vi "prepAI_tt.vi"   [LabVIEW 2013]
uses:
  <vilib>/DAQmx/create/channels.llb/DAQmx Create Channel (AI-Voltage-Basic).vi
  <vilib>/DAQmx/configure/timing.llb/DAQmx Timing (Sample Clock).vi
types:
  T1 = cluster{"StageS":i32, "StageL":i32, "data dir":path, "image OD":u16, "contour OD":u16, "point OD":u16, "AOlines":tag[], "AIlines":tag[], "CI lines":tag[], "DO lines":tag[], "AO names":string[], "CI names":string[], "AI names":string[], "DO names":string[], "CIextensions":string[], "AIextensions":string[], "Voltage to Ygalvo":i32, "Voltage to Xgalvo":i32, "Voltage to patch":i32, "640 shutter":i32, "2P shutter":i32, "LT timestamp":i32}
  T2 = typedef "LVRectTypeDef.ctl" = cluster{"Left":i16, "Top":i16, "Right":i16, "Bottom":i16}
  T3 = cluster{"Xpixels":i32, "Vxminref":dbl, "Vxmaxref":dbl, "P":dbl, "Ypixels":i32, "Vyminref":dbl, "Vymaxref":dbl, "srate":sgl, "sAOxy":i32, "timeout":dbl, "type":string, "date":string, "time":string, "Colormap":u16, "Drawing Mode":u16, "Scanning Mode":u16, "square pixels":bool, "square matrix":bool, "Xpixels Img":i32, "Vx-min Img":dbl, "VX-max Img":dbl, "Ypixels Img":i32, "Vy-min Img":dbl, "Vy-max Img ":dbl, "Angle Img":dbl, "autoshutter":bool, "finite":bool, "cont":bool, "wavdet":bool, "measpoints":i32, "avpp":i32, "bufferAO":i32, "bufferAI":i32, "starttick":u32, "waveform":path, "Vx-ref":dbl, "Vy-ref":dbl, "refreshrate":dbl, "refreshbuffer":i32, "tt_cycles":i32, "motorref":refnum<k7>, "mirrorswitch":refnum<k7>, "sample mode":i32, "maxbufferAI":i32, "sampletreshold":dbl, "srateAODO":sgl, "bin":sgl, "Pel":sgl, "Angle draw":dbl, "srate Img":sgl, "ROIimg_plotbounds":T2, "auto OD":bool, "ODfilt":u16, "reset AO_DO":bool, "aAI":i32[], "aCI":i32[], "aAO":i32[], "aDO":i32[]}
  T4 = cluster{" AI":refnum<k21>, "E_AI":errorcluster, "header":dbl[]}
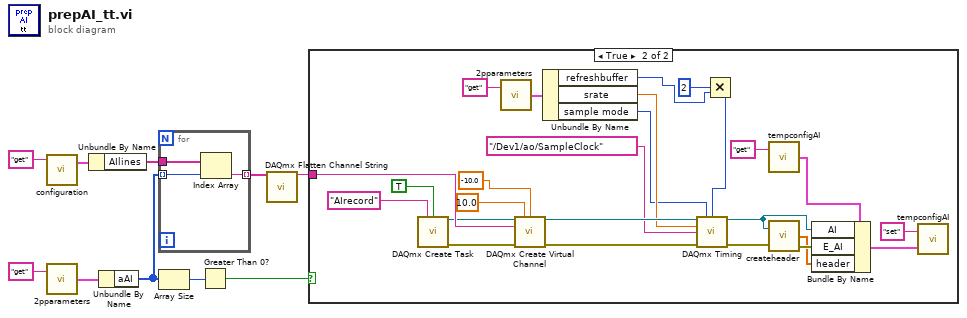
[diagram p0: block diagram]
diagram:
  n1 = call "configuration.vi"("command"="get") -> ("config out"=w7:T1)  [unwired: 2 in, 1 out]
  n2 = call "2pparameters.vi"("command"="get") -> ("params out"=w8:T3)  [unwired: 1 in]
  n3 = Unbundle By Name(w7) -> ("AIlines"=w6:tag[])
  n4 = Unbundle By Name(w8) -> ("aAI"=w4:i32[])
  n5 = for {
    tunnel: w4 -> [w13] mode=indexing
    tunnel: w6 -> [w12]
    tunnel: [w11] -> w5 mode=indexing
    n6 = Index Array(array=w12, index=w13) -> (element=w11:tag)
  }
  n7 = Array Size(array=w4) -> (size(s)=w3:i32)
  n8 = Greater Than 0?(x=w3) -> (x > 0?=w1:bool)
  n9 = call <vilib>:"DAQmx Flatten Channel String.vi"("names in"=w5) -> ("names out"=w2:string)  [unwired: 13 in, 1 out]
  n10 = case shown="True" w1 {
    tunnel: w2 -> [_ w34]
    frame False {
    }
    frame True {
      n11 = call <vilib>:"DAQmx Create Task.vi"("new task name"="AIrecord", "auto cleanup"=TRUE) -> ("task out"=w18:refnum<k21>, "error out"=w19:errorcluster)  [unwired: 12 in]
      n12 = call "2pparameters.vi"("command"="get") -> ("params out"=w36:T3)  [unwired: 1 in]
      n13 = call-poly <vilib>:"DAQmx Create Virtual Channel.vi"("task in"=w18, "maximum value"=10.0, "minimum value"=-10.0, "physical channels"=w34, "error in"=w19) -> ("task out"=w38:refnum<k21>, "error out"=w37:errorcluster)  [unwired: 9 in]
      n14 = Unbundle By Name(w36) -> ("refreshbuffer"=w15:i32, "srate"=w29:sgl, "sample mode"=w27:i32)
      n15 = Multiply(x=2, y=w15) -> (x*y=w14:i32)
      n16 = call-poly <vilib>:"DAQmx Timing.vi"("task/channels in"=w38, "sample mode"=w27, "samples per channel"=w14, "rate"=w29, "source"=tag "/Dev1/ao/SampleClock", "error in"=w37) -> ("task out"=w24:refnum<k21>, "error out"=w23:errorcluster)  [unwired: 8 in]
      n17 = call "tempconfigAI.vi"("command"="get") -> ("Temp Config out"=w32:T4)  [unwired: 1 in]
      n18 = call "createheader.vi"("task in"=w24, "error in"=w23) -> ("Array"=w21:dbl[], "error out"=w22:errorcluster)  [unwired: 1 out]
      n19 = Bundle By Name(cluster=w32, "AI"=w24, "E_AI"=w22, "header"=w21) -> (w33:T4)
      n20 = call "tempconfigAI.vi"("Temp Config in"=w33, "command"="set") -> ()  [unwired: 1 out]
    }
  }
